vi "Main.vi"() -> ()   [LabVIEW 2016]
doc: "This example reads data from Infrared Proximity Sensor, processes the data and displays the data on the waveform chart."
panel:
  out "Gauge":dbl(knob) scale=10.0..80.0
  out "error out":errorcluster
  out "Distance Waveform":dbl(graph)
  in  "Stop":bool
  in  "Calibration Parameters":cluster{"k":dbl, "b":dbl, "m":dbl}={"k"=1.8233599662780762, "b"=0.2962961196899414, "m"=0.17500019073486328}
  # "Overview: This example reads data from Infrared Proximity Sensor, processes the data and displays the data on the waveform chart. \nInstructions:\n1. Connect the sensor to myRIO.\n     GP2Y0A21YK0F                    myRIO\n      VCC                                         +5V\n      Gnd                                         Gnd\n      Vo                                            Connector A/AI0\n2. Check the myRIO target IP Address in the project and make sure the target IP Address is correct.\n3. Run this VI. The LED shows whether there are objects in the detection range( 0.1m - 0.8m)\n4. The Calibration Parameters are calculated using Calibration.vi."
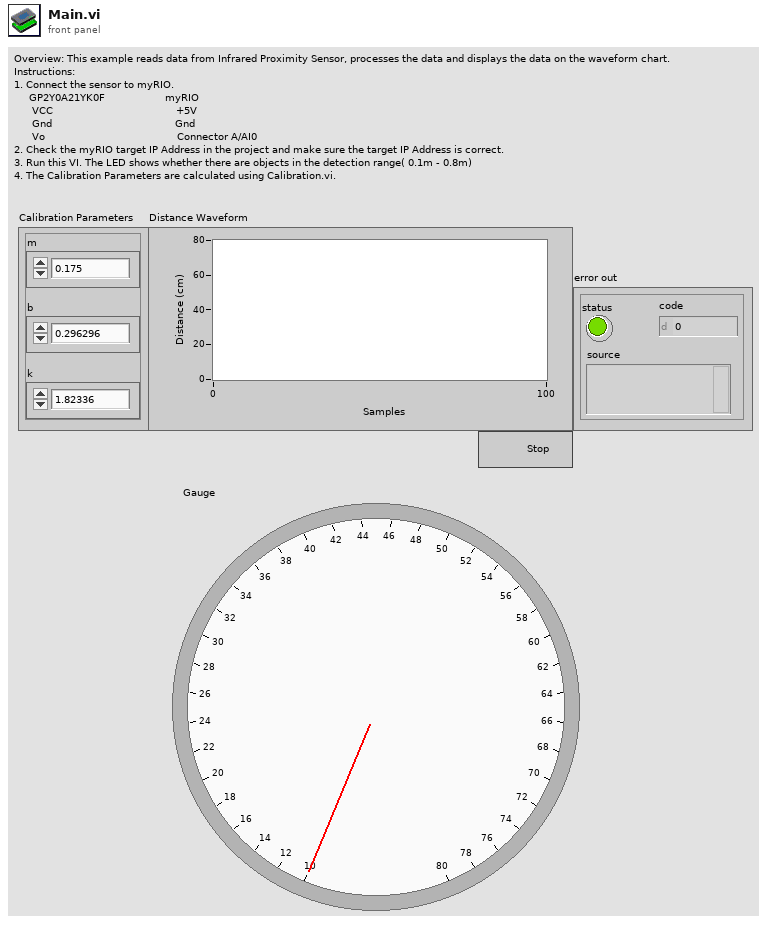
[diagram p1: front panel]
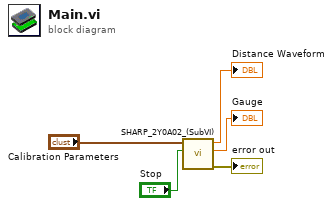
[diagram p0: block diagram]
diagram:
  n1 = call "SHARP_2Y0A02_(SubVI).vi"("Stop"="Stop", "Calibration Parameters"="Calibration Parameters") -> ("error out"=→"error out":errorcluster, "Gauge"=→"Gauge":dbl, "Distance Waveform"=→"Distance Waveform":dbl)  [unwired: 7 in]
